vi "PS FPGA Filter.vi"(9 "loop?":bool, 11 "input":fxp<+/-,20,5>[](array[numeric])=[0.0, 0.0, 0.0, 0.0, 0.0, 0.0, 0.0, 0.0]) -> (3 "output":fxp<+/-,20,5>[](array[numeric]))   [LabVIEW 2011]
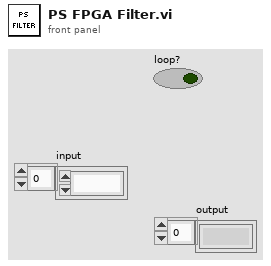
[diagram p1: front panel]
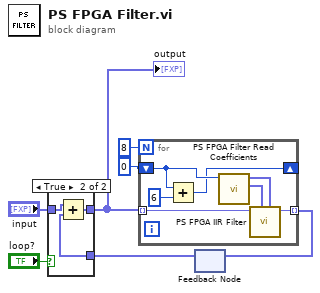
[diagram p0: block diagram]
diagram:
  n1 = feedback #1() -> (w6:fxp<+/-,20,5>[])  [unwired: 1 in]
  n2 = case shown="True" "loop?" {
    tunnel: [w8 w11] -> w1
    tunnel: w6 -> [_ w10]
    tunnel: "input" -> [w8 w9]
    frame False {
    }
    frame True {
      n3 = Add(x=w9, y=w10) -> (x+y=w11:fxp<+/-,20,5>[])
    }
  }
  "output" <- w1
  n4 = for {
    N: 8 -> [_]
    tunnel: w1 -> [w18] mode=indexing
    tunnel: [w17] -> w2 mode=indexing
    shift-right: [w12] -> _
    shift-left: u8 0 -> [w13]
    n5 = Add(x=w13, y=u8 6) -> (x+y=w12:u8)
    n6 = call "PS FPGA Filter Read Coefficients.vi"("offset"=w13) -> ("a coeffs"=w14:fxp<+/-,20,2>[], "b coeffs"=w15:fxp<+/-,20,2>[])  [unwired: 9 in]
    n7 = call "PS FPGA IIR Filter.vi"("coeff_b"=w15, "coeff_a"=w14, "input data"=w18) -> ("output data"=w17:fxp<+/-,20,5>)  [unwired: 8 in]
  }
  n8 = feedback-in #1(w2) -> ()
